vi "test_Create Global MetaData Channel_error on empty name.vi"(8 "error in (no error)":errorcluster, 11 "TestCase in":refnum<class "Instrument Addon Scripting API Channels Unit Tests.lvclass">) -> (0 "error out":errorcluster, 3 "TestCase out":refnum<class "Instrument Addon Scripting API Channels Unit Tests.lvclass">)   [LabVIEW 2018, in "Instrument Addon Scripting API Channels Unit Tests.lvclass"]
uses:
  Instrument Addon Scripting API Channels Unit Tests.lvclass
  APIs/Scripting API/TypeDefs/Array Type Cast Settings.ctl
  APIs/Scripting API/TypeDefs/Array Element.ctl
  Addon/Addon Shared/Types/Type Cast Type.ctl
  Addon/Addon Shared/Types/Endian.ctl
  Instrument Addon Scripting API Channels Unit Tests.lvclass/Instrument Addon Scripting API Channels Unit Tests.ctl
  APIs/Scripting API/Channels/Create Global MetaData Channel - Array - Type Cast.vi
  <vilib>/addons/_JKI Toolkits/VI Tester/TestCase.llb/TestCase.lvclass
  Instrument Addon Scripting API Test Assets/Instrument Addon Scripting API Test Assets.lvclass
  APIs/Scripting API/Instrument Addon Scripting API.lvlib
  Addon/Addon Shared/Instrument Addon Shared.lvlib
  C:/Program Files (x86)/National Instruments/LabVIEW 2018/vi.lib/addons/_JKI Toolkits/VI Tester/TestCase.llb/TestCase.lvclass
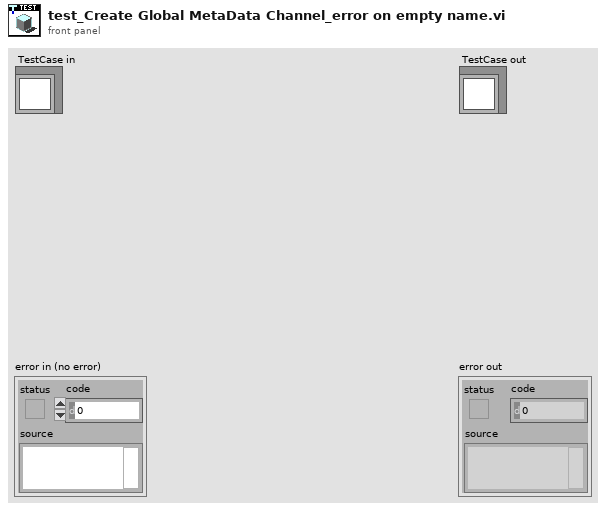
[diagram p1: front panel]
types:
  T1 = typedef "Instrument Addon Scripting API.lvlib/Array Type Cast Settings.ctl" = cluster{"Elements":T2[], "Type":T3, "Endian":T4, "Delimiter":string}
  T2 = typedef "Instrument Addon Scripting API.lvlib/Array Element.ctl" = cluster{"Name":string, "Default Value":dbl, "Units":string}
  T3 = typedef "Instrument Addon Shared.lvlib/Type Cast Type.ctl" = enum16{"DBL", "SGL", "U64", "U32", "U16", "U8", "I64", "I32", "I16", "I8"}
  T4 = typedef "Instrument Addon Shared.lvlib/Endian.ctl" = enum16{"Native", "Little", "Big"}
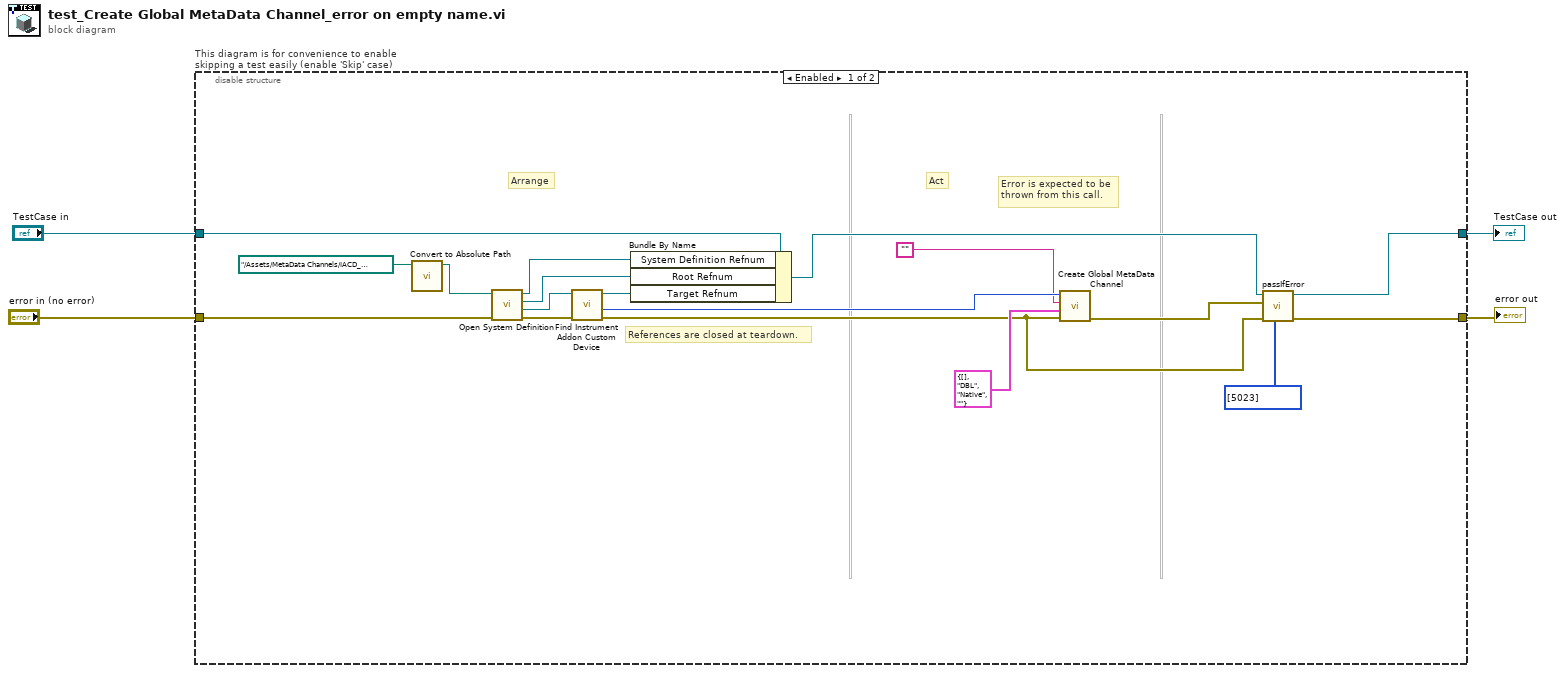
[diagram p0: block diagram]
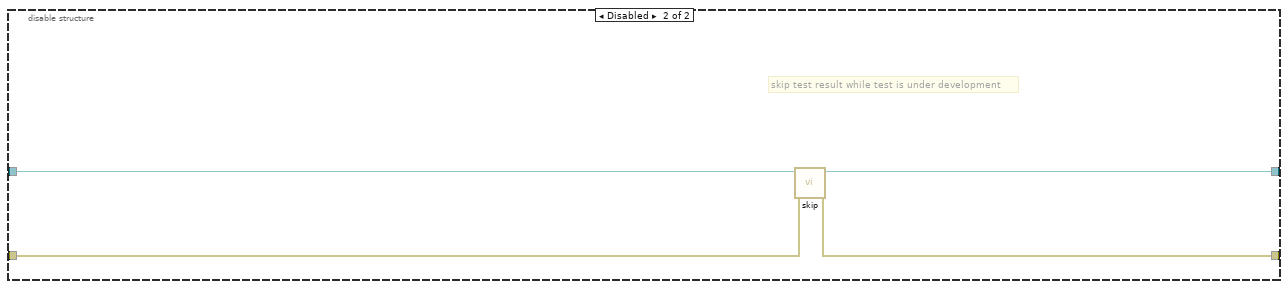
[diagram p2: hidden frame]
diagram:
  n1 = disable-structure "This diagram is for convenience to enable skipping a test easily (enable 'Skip' case)" shown="Enabled" {
    disable-tunnel: "TestCase in" -> [w16 w26]
    disable-tunnel: [w15 w24] -> w1
    disable-tunnel: [w14 w25] -> w3
    disable-tunnel: "error in (no error)" -> [w22 w23]
    frame Enabled {
      # "Error is expected to be\nthrown from this call."
      # "References are closed at teardown."
      # "Act"
      # "Arrange"
      n2 = call "Convert to Absolute Path.vi"("System Definition File"=path "../Assets/MetaData Channels/IACD_channels.nivssdf") -> ("Absolute Path"=w5:path)  [unwired: 10 in]
      n3 = call "Open System Definition.vi"("error in (no error)"=w22, "System Definition File"=w5) -> ("error out"=w20:errorcluster, "Target Refnum"=w21:refnum<k24>, "Root Refnum"=w18:refnum<k24>, "System Definition Refnum"=w17:refnum<k24>)  [unwired: 6 in]
      n4 = call "Find Instrument Addon Custom Device.vi"("error in"=w20, "target in"=w21) -> ("error out"=w9:errorcluster, "NodeID"=w8:u64, "target out"=w19:refnum<k24>)  [unwired: 7 in]
      n5 = Bundle By Name(cluster=w16, "System Definition Refnum"=w17, "Root Refnum"=w18, "Target Refnum"=w19) -> (w12:refnum<class "Instrument Addon Scripting API Channels Unit Tests.lvclass">)
      n6 = call-poly "Create Global MetaData Channel.vi"("Error In"=w9, "Settings"=T1 {"Elements"=[], "Type"=enum."DBL", "Endian"=enum."Native", "Delimiter"=""}, "Name"="", "Instrument Addon Refnum In"=w8) -> ("Error Out"=w10:errorcluster)  [unwired: 4 in, 3 out]
      n7 = call-dynamic "passIfError.vi"("passing error codes (default = any error code)"=i32[] [5023], "error in (no error)"=w9, "error"=w10, "TestCase in"=w12) -> ("error out"=w14:errorcluster, "TestCase out"=w15:refnum<class "Instrument Addon Scripting API Channels Unit Tests.lvclass">)  [unwired: 6 in]
    }
    frame Disabled {
      # "skip test result while test is under development"
      n8 = call <vilib>:"skip.vi"("error in (no error)"=w23, "TestCase in"=w26) -> ("error out"=w25:errorcluster, "TestCase out"=w24:refnum<class "Instrument Addon Scripting API Channels Unit Tests.lvclass">)  [unwired: 8 in]
    }
  }
  "error out" <- w3
  "TestCase out" <- w1
